vi "switchRelays.vi"(8 "error in":errorcluster, 11 "controlRelays":u8) -> (0 "error out":errorcluster, 3 "debugControlRelays":u8)   [LabVIEW 2018]
doc: "Takes the numeric input value of <b>controlRelay</b> and sends it to the cRIO module, using the FPGA I/O Node."
uses:
  <vilib>/rvi/eio/common/nirviEmuTemplateMethod_errors.vi
  <vilib>/eio/EIONode/EIONode.xnode
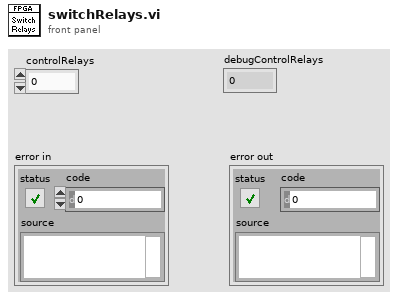
[diagram p1: front panel]
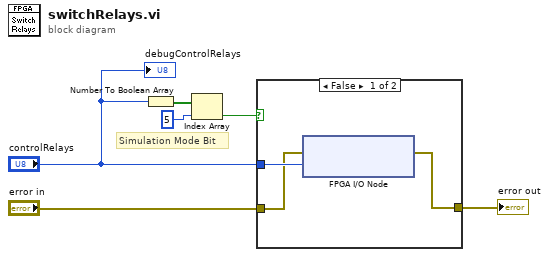
[diagram p0: block diagram]
diagram:
  # "Simulation Mode Bit"
  n1 = Number To Boolean Array(number="controlRelays") -> (Boolean array=w5:bool[])
  n2 = Index Array(array=w5, index=5) -> (element=w3:bool)
  n3 = case shown="False" w3 {
    tunnel: "controlRelays" -> [w9 _]
    tunnel: [w8 w10] -> w2
    tunnel: "error in" -> [w7 w10]
    frame False {
      n4 = xnode "FPGA I/O Node"("error in"=w7, "Mod4/CH7:0"=w9) -> ("error out"=w8:errorcluster)  [unwired: 1 in, 1 out]
    }
    frame True {
      # "In here there will be \na simulation code"
      # "Simulation Mode On"
    }
  }
  "error out" <- w2
  "debugControlRelays" <- "controlRelays"
